vi "Add Active DUT Connector.vi"(8 "error in (no error)":errorcluster, 10 "Connector Name (\"Connector1\")":string="Connector1", 11 "VISA resource name":refnum<visa-resource-name>) -> (0 "error out":errorcluster, 3 "VISA resource name out":refnum<visa-resource-name>)   [LabVIEW 2020, in "Rohde&Schwarz CMXP Base.lvlib"]
doc: "Creates an antenna connector for the active DUT.\n\nAssign a unique name to each named object within the test environment. Assigning an already used name can be rejected with an error message, even if the other object has not the same type as the new object.\n\nAttribute:\nRSCMXPBASE_ATTR_ACTIVE_DUT_CONNECTOR_ADD\n\nRemote-control command:\nCREate:DUT:CONNector"
uses:
  <instrlib>/Rohde&Schwarz CMXP Base/Rohde&Schwarz CMXP Base.lvlib
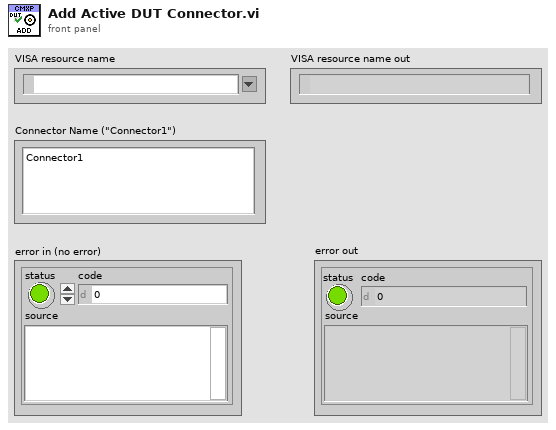
[diagram p1: front panel]
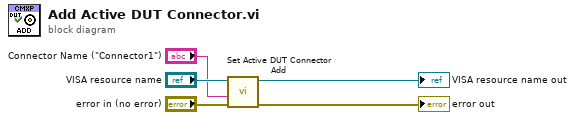
[diagram p0: block diagram]
diagram:
  n1 = call "Set Active DUT Connector Add"("error in (no error)"="error in (no error)", "Active DUT Connector Add ()"="Connector Name (\"Connector1\")", "instrument handle"="VISA resource name") -> ("error out"=→"error out":errorcluster, "instrument handle out"=→"VISA resource name out":refnum<visa-resource-name>)  [unwired: 7 in]
